vi "TCP-IP Q_Bridge.Core.vi"(4 "Notification":bool, 6 "Auto Exit":bool, 7 "StatusCtrlRef":refnum<vi>, 8 "Config":T1={"IP"="127.0.0.1", "Port"=8500, "Listener"=FALSE, "Enable"=FALSE}, 9 "Q_DataOut":refnum<queue> caption="Q_DataOut(To TCP-IP)", 10 "Q_DataIn":refnum<queue> caption="Q_DataIn(From TCP-IP)", 11 "Control Q":string="TCP-IP_Bridge") -> ()   [LabVIEW 2024, in "EQMF.lvlib" / "TCP-IP.lvlib"]
uses:
  TCP-IP.lvlib
  Queues/Q.Element.ctl
  Mgr/TCP-IP Mgr.Config.ctl
  Queues/Queue Utils.lvlib
panel:
  out "Close":bool
  out "connection ID":refnum<k5>
  out "listener ID":refnum<k5>
  out "Exit":bool
  out "Connected":bool
  out "error out":errorcluster
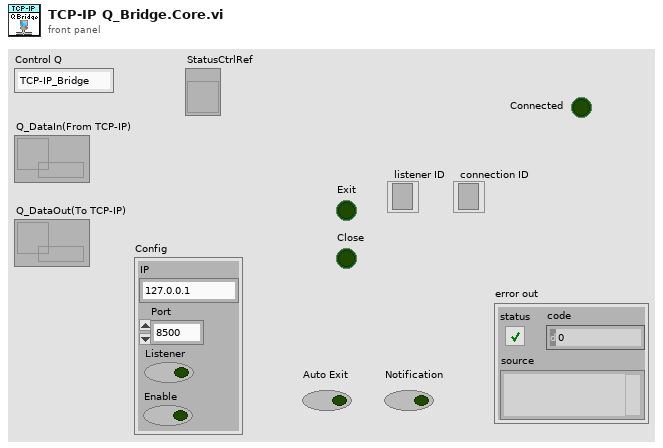
[diagram p1: front panel]
types:
  T1 = typedef "EQMF.lvlib/TCP-IP.lvlib/TCP-IP Mgr.Config.ctl" = cluster{"IP":string, "Port":u16, "Listener":bool, "Enable":bool}
  T2 = typedef "EQMF.lvlib/Queue Utils.lvlib/Q.Element.ctl" = cluster{"Cmd":string, "Sub":string, "Data1":variant, "Data2":variant}
  T3 = cluster{"Config":T1, "ConnectionID":refnum<k5>, "listenerID":refnum<k5>, "Connected":bool, "StatusCtrlRef":refnum<vi>, "CtrlRefEn":bool}
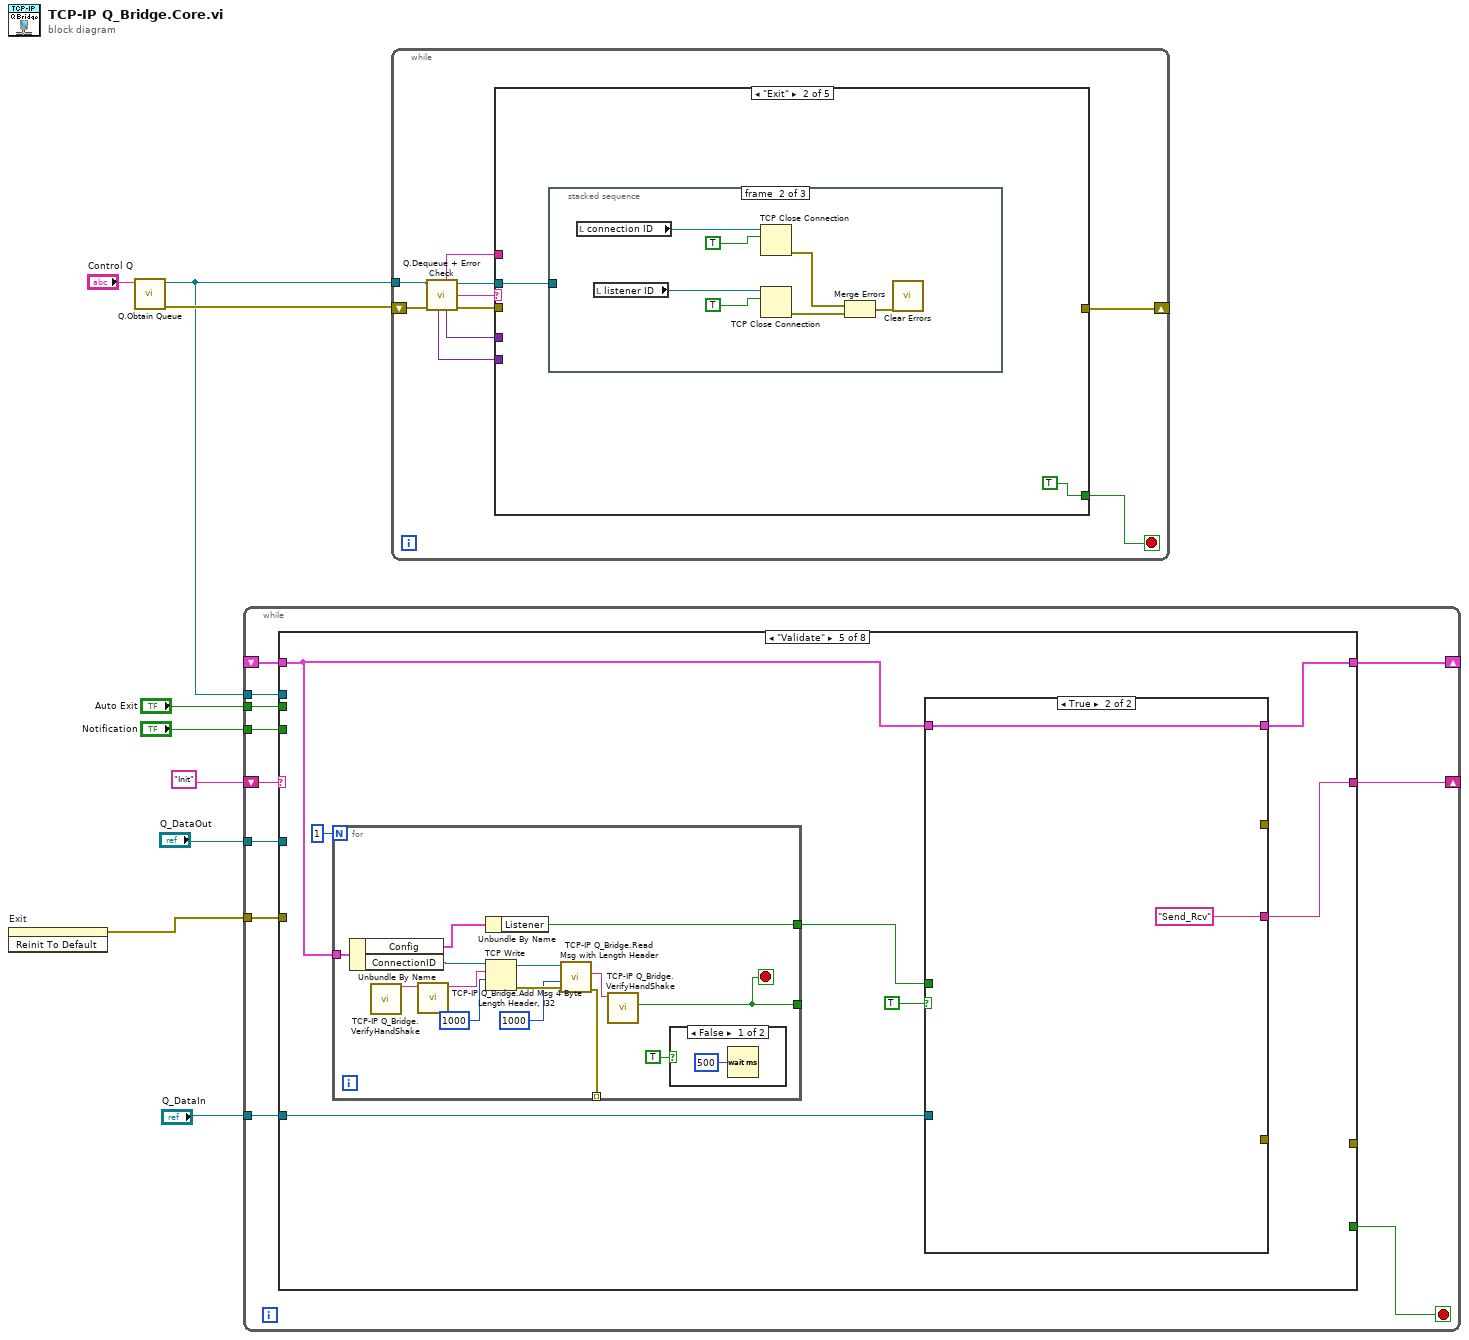
[diagram p0: block diagram]
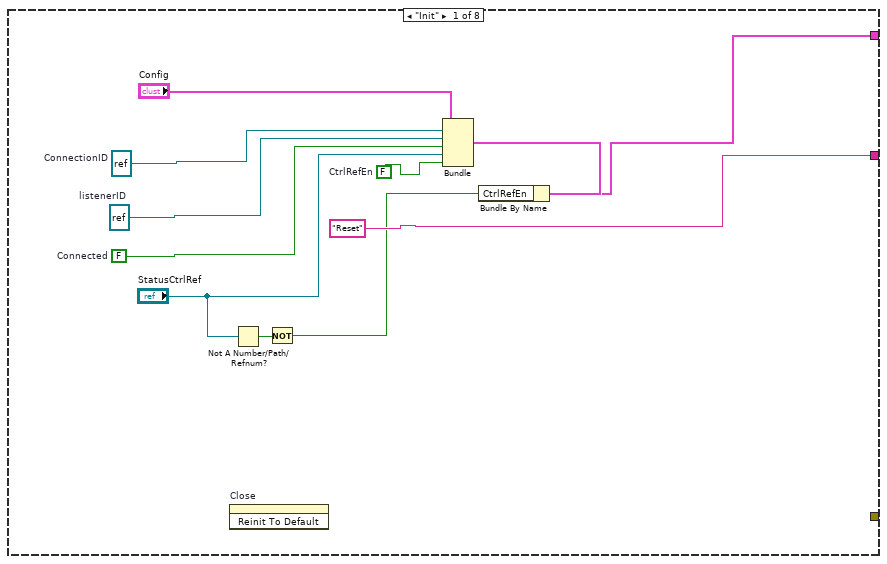
[diagram p2: hidden frame]
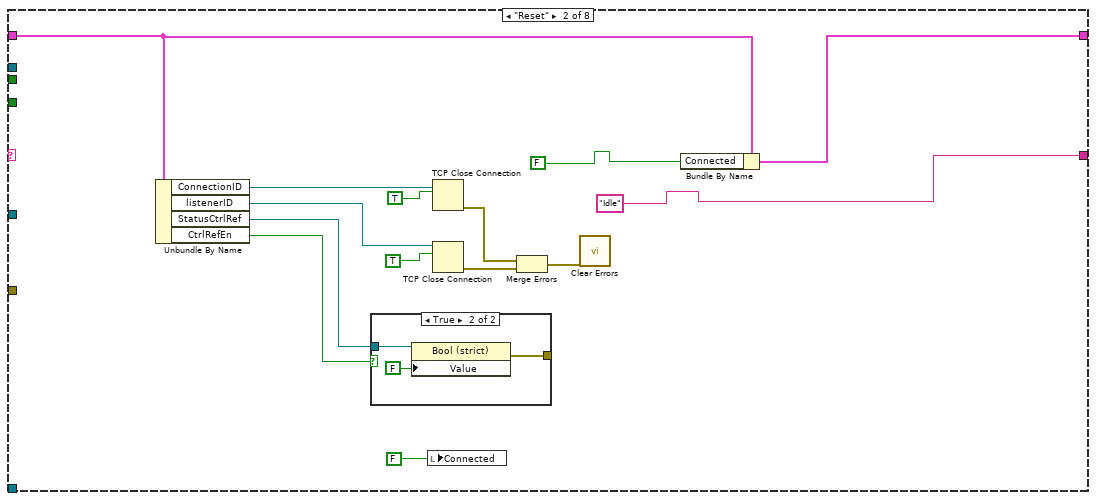
[diagram p3: hidden frame]
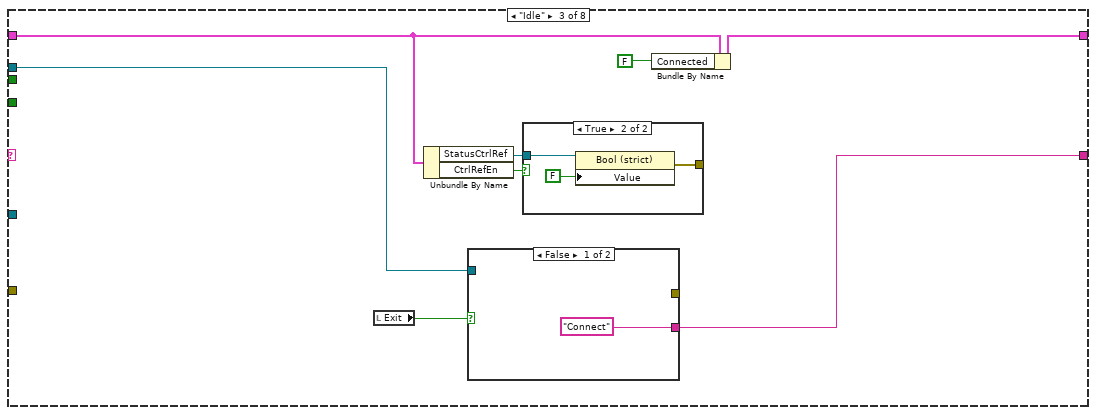
[diagram p5: hidden frame]
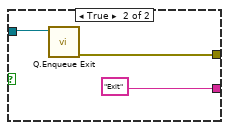
[diagram p7: hidden frame]
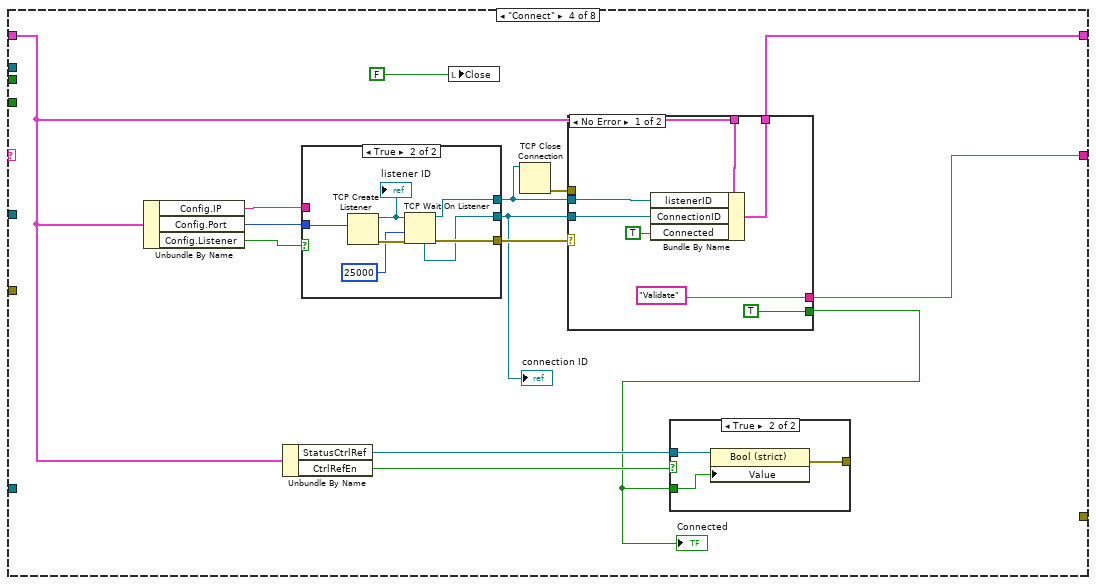
[diagram p8: hidden frame]
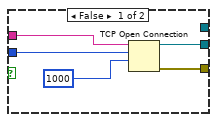
[diagram p10: hidden frame]
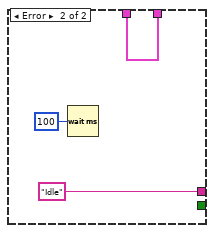
[diagram p11: hidden frame]
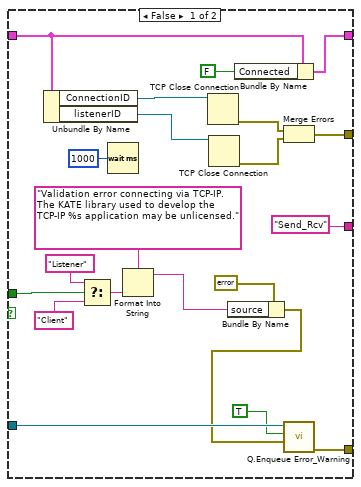
[diagram p13: hidden frame]
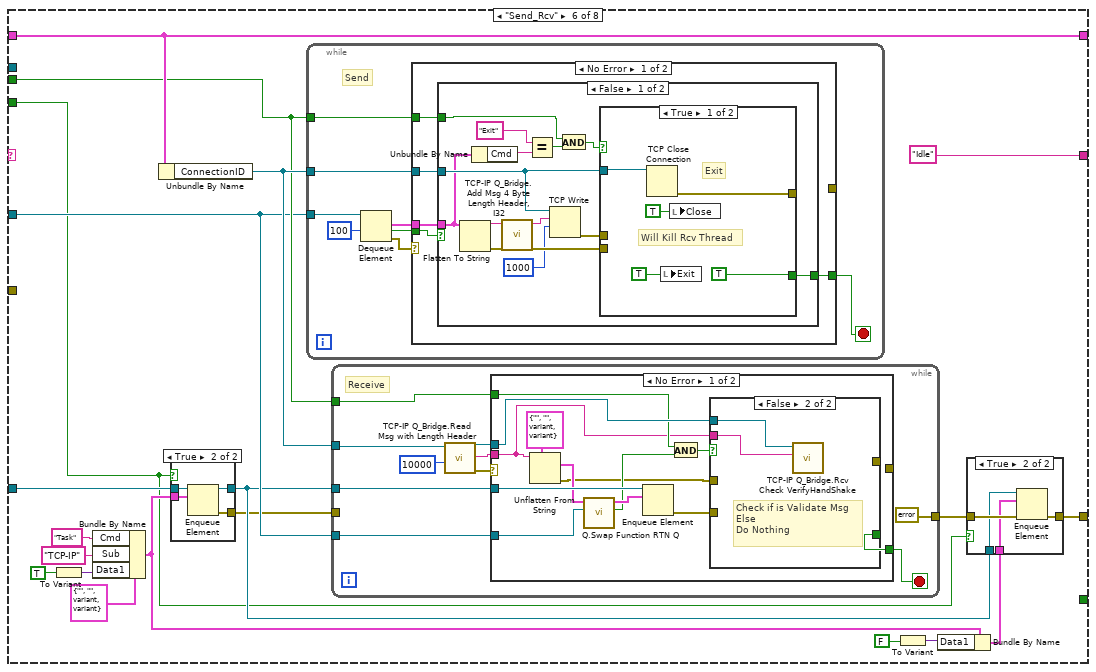
[diagram p14: hidden frame]
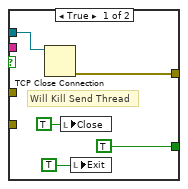
[diagram p17: hidden frame]
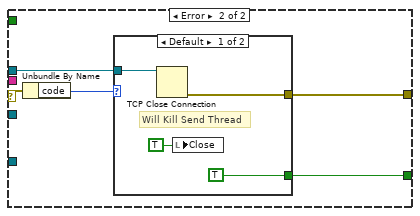
[diagram p18: hidden frame]
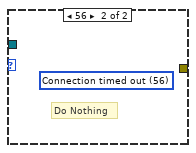
[diagram p19: hidden frame]
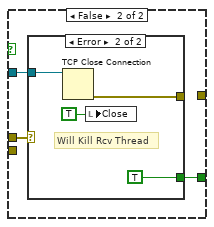
[diagram p20: hidden frame]
diagram:
  n1 = invoke on="Exit" class="Bool (strict)" method="Reinit To Default"() -> (error out=w4:errorcluster)  [unwired: 3 in, 2 out]
  n2 = call "Q.Obtain Queue.vi"("Q Name"="Control Q") -> ("error out"=w8:errorcluster, "Q Out"=w3:refnum<queue>)  [unwired: 8 in, 1 out]
  n3 = while {
    shift-right: [w18] -> _
    shift-left: _ -> [w19]
    shift-right: [w13] -> _
    shift-left: "Init" -> [w20]
    tunnel: "Q_DataOut" -> [w16]
    tunnel: "Q_DataIn" -> [w15]
    tunnel: w4 -> [w14]
    tunnel: w3 -> [w12]
    tunnel: "Auto Exit" -> [w11]
    tunnel: "Notification" -> [w10]
    stop <- w17 stop-if-true
    n4 = case shown="\"Validate\"" w20 {
      tunnel: w19 -> [_ w38 w51 w70 w107 w167 w262 w270]
      tunnel: [w22 w37 w56 w75 w106 w167 w262 w270] -> w18
      tunnel: ["Reset" "Idle" w54 w74 w109 "Idle" "Reset" "Exit"] -> w13
      tunnel: [_ _ _ _ _ _ _ TRUE] -> w17
      tunnel: w16 -> [_ _ _ _ _ w163 _ _]
      tunnel: w15 -> [_ _ _ _ w105 w157 _ _]
      tunnel: w14 -> [_ _ _ _ _ _ _ _]
      tunnel: w12 -> [_ _ w52 _ _ _ _ w265]
      tunnel: w11 -> [_ _ _ _ _ w164 _ _]
      tunnel: w10 -> [_ _ _ _ _ w148 _ _]
      tunnel: [_ _ _ _ _ w155 _ _] -> _
      frame "Init" {
        w24 = FALSE  # CtrlRefEn
        w27 = FALSE  # Connected
        w28 = refnum<k5> refnum  # listenerID
        w29 = refnum<k5> refnum  # ConnectionID
        n5 = invoke on="Close" class="Bool (strict)" method="Reinit To Default"() -> ()  [unwired: 3 in, 3 out]
        n6 = Not A Number/Path/Refnum?(number/path/refnum="StatusCtrlRef") -> (NaN/Path/Refnum?=w25:bool)
        n7 = Not(x=w25) -> (.not. x?=w21:bool)
        n8 = Bundle("Config"="Config", "ConnectionID"=w29, "listenerID"=w28, "Connected"=w27, "StatusCtrlRef"="StatusCtrlRef", "CtrlRefEn"=w24) -> (w23:T3)  [unwired: 1 in]
        n9 = Bundle By Name(cluster=w23, "CtrlRefEn"=w21) -> (w22:T3)
      }
      frame "Reset" {
        n10 = Unbundle By Name(w38) -> ("ConnectionID"=w45:refnum<k5>, "listenerID"=w42:refnum<k5>, "StatusCtrlRef"=w34:refnum<vi>, "CtrlRefEn"=w33:bool)
        n11 = case shown="True" w33 {
          tunnel: w34 -> [_ w48]
          tunnel: [_ w46] -> _
          frame False {
          }
          frame True {
            n12 = property class="Bool (strict)"(reference=w48, "Value"=FALSE) -> (error out=w46:errorcluster)  [unwired: 1 in, 1 out]
          }
        }
        n13 = local write "Connected"(FALSE ("Value")) -> ()
        n14 = TCP Close Connection(connection ID=w45, abort (F)=TRUE) -> (error out=w40:errorcluster)  [unwired: 1 in, 1 out]
        n15 = TCP Close Connection(connection ID=w42, abort (F)=TRUE) -> (error out=w41:errorcluster)  [unwired: 1 in, 1 out]
        n16 = Merge Errors(w40, w41) -> (w39:errorcluster)
        n17 = call <vilib>:"Clear Errors.vi"("error in (no error)"=w39) -> ()  [unwired: 5 in, 2 out]
        n18 = Bundle By Name(cluster=w38, "Connected"=FALSE) -> (w37:T3)
      }
      frame "Idle" {
        n19 = local read "Exit"() -> (w53:bool)
        n20 = Unbundle By Name(w51) -> ("StatusCtrlRef"=w50:refnum<vi>, "CtrlRefEn"=w49:bool)
        n21 = case shown="False" w53 {
          tunnel: ["Connect" "Exit"] -> w54
          tunnel: w52 -> [_ w62]
          tunnel: [_ w61] -> _
          frame False {
          }
          frame True {
            n22 = call "Q.Enqueue Exit.vi"("Q In"=w62) -> ("error out"=w61:errorcluster)  [unwired: 9 in, 1 out]
          }
        }
        n23 = case shown="True" w49 {
          tunnel: w50 -> [_ w59]
          tunnel: [_ w58] -> _
          frame False {
          }
          frame True {
            n24 = property class="Bool (strict)"(reference=w59, "Value"=FALSE ("Connected")) -> (error out=w58:errorcluster)  [unwired: 1 in, 1 out]
          }
        }
        n25 = Bundle By Name(cluster=w51, "Connected"=FALSE) -> (w56:T3)
      }
      frame "Connect" {
        n26 = Unbundle By Name(w70) -> ("Config.IP"=w77:string, "Config.Port"=w76:u16, "Config.Listener"=w72:bool)
        n27 = Unbundle By Name(w70) -> ("StatusCtrlRef"=w69:refnum<vi>, "CtrlRefEn"=w68:bool)
        n28 = case shown="True" w72 {
          tunnel: w77 -> [w85 _]
          tunnel: w76 -> [w84 w92]
          tunnel: [w82 w87] -> w71
          tunnel: [w81 w89] -> w73
          tunnel: [_ w88] -> w65
          frame False {
            n29 = TCP Open Connection(address=w85, remote port or service name=w84, timeout ms (60000)=1000) -> (connection ID=w82:refnum<k5>, error out=w81:errorcluster)  [unwired: 2 in]
          }
          frame True {
            n30 = TCP Create Listener(10:w92) -> (0:w91:errorcluster, 3:w90:refnum<k5>)  [unwired: 4 in, 1 out]
            "listener ID" <- w90
            n31 = TCP Wait On Listener(8:w91, 9:25000 ("timeout ms (wait forever: -1)"), 11:w90) -> (0:w89:errorcluster, 3:w88:refnum<k5>, 4:w87:refnum<k5>)  [unwired: 1 in, 2 out]
          }
        }
        "connection ID" <- w71
        n32 = local write "Close"(FALSE ("Reset")) -> ()
        n33 = TCP Close Connection(connection ID=w65) -> (error out=w64:errorcluster)  [unwired: 2 in, 1 out]
        n34 = case shown="No Error" w73 {
          tunnel: w70 -> [w99 w100]
          tunnel: w71 -> [w97 _]
          tunnel: [w96 w100] -> w75
          tunnel: ["Validate" "Idle"] -> w74
          tunnel: w65 -> [w93 _]
          tunnel: [TRUE _] -> w67
          tunnel: w64 -> [_ _]
          frame No Error {
            n35 = Bundle By Name(cluster=w99, "listenerID"=w93, "ConnectionID"=w97, "Connected"=TRUE) -> (w96:T3)
          }
          frame Error {
            n36 = Wait (ms)(milliseconds to wait=u32 100) -> ()  [unwired: 1 out]
          }
        }
        "Connected" <- w67
        n37 = case shown="True" w68 {
          tunnel: w69 -> [_ w80]
          tunnel: [_ w79] -> _
          tunnel: w67 -> [_ w78]
          frame False {
          }
          frame True {
            n38 = property class="Bool (strict)"(reference=w80, "Value"=w78) -> (error out=w79:errorcluster)  [unwired: 1 in, 1 out]
          }
        }
      }
      frame "Validate" {
        n39 = for {
          N: 1 -> [_]
          tunnel: [w112] -> _
          tunnel: [w114] -> w108
          tunnel: w107 -> [w113]
          tunnel: [w111] -> _ mode=indexing
          stop <- w112 stop-if-true
          n40 = Unbundle By Name(w113) -> ("Config"=w115:T1, "ConnectionID"=w122:refnum<k5>)
          n41 = call "TCP-IP Q_Bridge.VerifyHandShake.vi"() -> ("Msg Out"=w117:string)  [unwired: 10 in, 1 out]
          n42 = call "TCP-IP Q_Bridge.Add Msg 4 Byte Length Header, I32.vi"("Message"=w117) -> ("Message + Header"=w123:string)  [unwired: 10 in]
          n43 = Unbundle By Name(w115) -> ("Listener"=w114:bool)
          n44 = TCP Write(connection ID=w122, data in=w123, 9:1000 ("timeout ms (25000)")) -> (connection ID out=w121:refnum<k5>, error out=w120:errorcluster)  [unwired: 1 in, 1 out]
          n45 = call "TCP-IP Q_Bridge.Read Msg with Length Header.vi"("error in (no error)"=w120, "Timeoutms"=1000 ("timeout ms (25000)"), "ConID"=w121) -> ("Error Out"=w111:errorcluster, "data out"=w116:string)  [unwired: 5 in, 2 out]
          n46 = call "TCP-IP Q_Bridge.VerifyHandShake.vi"("Msg In"=w116) -> ("OK"=w112:bool)  [unwired: 9 in, 1 out]
          n47 = case shown="False" TRUE {
            frame False {
              n48 = Wait (ms)(milliseconds to wait=u32 500) -> ()  [unwired: 1 out]
            }
            frame True {
            }
          }
        }
        n49 = case shown="True" TRUE {
          tunnel: ["Send_Rcv" "Send_Rcv"] -> w109
          tunnel: w108 -> [w142 _]
          tunnel: w107 -> [w136 w146]
          tunnel: [w137 w146] -> w106
          tunnel: [w131 _] -> _
          tunnel: w105 -> [w130 _]
          tunnel: [w125 _] -> _
          frame False {
            n50 = Unbundle By Name(w136) -> ("ConnectionID"=w135:refnum<k5>, "listenerID"=w134:refnum<k5>)
            n51 = Select(t="Listener", s=w142, f="Client") -> (s? t:f=w143:string)
            n52 = Wait (ms)(milliseconds to wait=u32 1000) -> ()  [unwired: 1 out]
            n53 = Format Into String(format string="Validation error connecting via TCP-IP.  The KATE library used to develop the TCP-IP %s application may be unlicensed." ("message"), w143) -> (resulting string=w128:string)  [unwired: 2 in, 1 out]
            n54 = TCP Close Connection(connection ID=w135) -> (error out=w133:errorcluster)  [unwired: 2 in, 1 out]
            n55 = TCP Close Connection(connection ID=w134) -> (error out=w132:errorcluster)  [unwired: 2 in, 1 out]
            n56 = Bundle By Name(cluster=errorcluster {"status"=TRUE, "code"=-8000, "source"=""} ("error constant"), "source"=w128) -> (w127:errorcluster)
            n57 = Bundle By Name(cluster=w136, "Connected"=FALSE) -> (w137:T3)
            n58 = Merge Errors(w133, w132) -> (w131:errorcluster)
            n59 = call "Q.Enqueue Error_Warning.vi"("Error/Warning"=w127, "Warning(F)/Error(T)"=TRUE, "Q In"=w130) -> ("error out"=w125:errorcluster)  [unwired: 7 in, 1 out]
          }
          frame True {
          }
        }
      }
      frame "Send_Rcv" {
        n60 = To Variant(anything=TRUE) -> (Variant=w161:variant)
        n61 = Bundle By Name(cluster=T2 {"Cmd"="", "Sub"="", "Data1"=variant, "Data2"=variant} ("Q.Element"), "Cmd"="Task", "Sub"="TCP-IP", "Data1"=w161) -> (w151:T2)
        n62 = Unbundle By Name(w167) -> ("ConnectionID"=w166:refnum<k5>)
        n63 = case shown="True" w148 {
          tunnel: w157 -> [w172 w176]
          tunnel: [w172 w175] -> w154
          tunnel: w151 -> [_ w174]
          tunnel: [_ w173] -> w149
          frame False {
          }
          frame True {
            n64 = Enqueue Element(queue=w176, element=w174) -> (queue out=w175:refnum<queue>, error out=w173:errorcluster)  [unwired: 2 in, 1 out]
          }
        }
        n65 = while {
          tunnel: w163 -> [w222]
          tunnel: w166 -> [w220]
          tunnel: w164 -> [w217]
          stop <- w223 stop-if-true
          # "Send"
          n66 = Dequeue Element(queue=w222, timeout in ms (-1)=100) -> (element=w218:T2, timed out?=w219:bool, error out=w216:errorcluster)  [unwired: 1 in, 1 out]
          n67 = case shown="No Error" w216 {
            tunnel: [w228 TRUE] -> w223
            tunnel: w220 -> [w227 w257]
            tunnel: w219 -> [w226 _]
            tunnel: w218 -> [w225 _]
            tunnel: w217 -> [w224 _]
            tunnel: [_ w256] -> _
            frame No Error {
              n68 = case shown="False" w226 {
                tunnel: [w241 w254] -> w228
                tunnel: w225 -> [w238 _]
                tunnel: w227 -> [w240 _]
                tunnel: w224 -> [w233 _]
                frame False {
                  n69 = Flatten To String(anything=w238) -> (data string=w232:string, error out=w230:errorcluster)  [unwired: 3 in, 1 out]
                  n70 = Unbundle By Name(w238) -> ("Cmd"=w237:string)
                  n71 = call "TCP-IP Q_Bridge.Add Msg 4 Byte Length Header, I32.vi"("Message"=w232) -> ("Message + Header"=w231:string)  [unwired: 10 in]
                  n72 = Equal?(x="Exit", y=w237) -> (x = y?=w235:bool)
                  n73 = TCP Write(connection ID=w240, data in=w231, 9:1000 ("timeout ms (25000)")) -> (error out=w239:errorcluster)  [unwired: 1 in, 2 out]
                  n74 = And(x=w233, y=w235) -> (x .and. y?=w234:bool)
                  n75 = case shown="True" w234 {
                    tunnel: [TRUE w249] -> w241
                    tunnel: w240 -> [w245 w248]
                    tunnel: w239 -> [_ w247]
                    tunnel: [w244 _] -> _
                    tunnel: w230 -> [_ _]
                    frame True {
                      # "Exit"
                      # "Will Kill Rcv Thread"
                      n76 = TCP Close Connection(connection ID=w245) -> (error out=w244:errorcluster)  [unwired: 2 in, 1 out]
                      n77 = local write "Exit"(TRUE ("Close")) -> ()
                      n78 = local write "Close"(TRUE ("Close")) -> ()
                    }
                    frame False {
                      n79 = case shown="Error" w247 {
                        tunnel: w248 -> [_ w252]
                        tunnel: [_ TRUE] -> w249
                        tunnel: [_ w251] -> _
                        frame No Error {
                        }
                        frame Error {
                          # "Will Kill Rcv Thread"
                          n80 = TCP Close Connection(connection ID=w252) -> (error out=w251:errorcluster)  [unwired: 2 in, 1 out]
                          n81 = local write "Close"(TRUE ("Close")) -> ()
                        }
                      }
                    }
                  }
                }
                frame True {
                  # "This time out allows ability to stop/exit"
                  # "Do nothing\nTimed Out"
                  n82 = local read "Close"() -> (w254:bool)
                }
              }
            }
            frame Error {
              # "Exit"
              # "Will Kill Rcv Thread"
              n83 = TCP Close Connection(connection ID=w257) -> (error out=w256:errorcluster)  [unwired: 2 in, 1 out]
              n84 = local write "Exit"(TRUE ("Close")) -> ()
              n85 = local write "Close"(TRUE ("Close")) -> ()
            }
          }
        }
        n86 = while {
          tunnel: w154 -> [w186]
          tunnel: w166 -> [w181]
          tunnel: w164 -> [w184]
          tunnel: w163 -> [w183]
          tunnel: [errorcluster {"status"=FALSE, "code"=0, "source"=""} ("error constant")] -> w156
          tunnel: w149 -> [_]
          stop <- w185 stop-if-true
          # "Receive"
          n87 = call "TCP-IP Q_Bridge.Read Msg with Length Header.vi"("Timeoutms"=10000 ("timeout ms (25000)"), "ConID"=w181) -> ("Error Out"=w178:errorcluster, "data out"=w179:string, "ConID Out"=w182:refnum<k5>)  [unwired: 6 in, 1 out]
          n88 = case shown="No Error" w178 {
            selector: w178 -> [_ w208]
            tunnel: w186 -> [w198 _]
            tunnel: w182 -> [w197 w210]
            tunnel: [w196 w211] -> w185
            tunnel: [_ w209] -> _
            tunnel: w184 -> [w194 _]
            tunnel: w183 -> [w190 _]
            tunnel: w179 -> [w187 _]
            frame No Error {
              n89 = Unflatten From String(type=T2 {"Cmd"="", "Sub"="", "Data1"=variant, "Data2"=variant} ("Q.Element"), binary string=w187) -> (value=w193:T2, error out=w189:errorcluster)  [unwired: 3 in, 1 out]
              n90 = call "Q.Swap Function RTN Q.vi"("RtnQ In"=w190, "Q.Element"=w193) -> ("Exit"=w191:bool, "Q.Element Out"=w192:T2)  [unwired: 8 in]
              n91 = Enqueue Element(queue=w198, element=w192) -> (error out=w188:errorcluster)  [unwired: 2 in, 2 out]
              n92 = And(x=w194, y=w191) -> (x .and. y?=w195:bool)
              n93 = case shown="False" w195 {
                tunnel: [TRUE _] -> w196
                tunnel: w197 -> [w203 w206]
                tunnel: [w202 _] -> _
                tunnel: w189 -> [_ _]
                tunnel: w188 -> [_ _]
                tunnel: w187 -> [_ w205]
                frame True {
                  # "Will Kill Send Thread"
                  n94 = TCP Close Connection(connection ID=w203) -> (error out=w202:errorcluster)  [unwired: 2 in, 1 out]
                  n95 = local write "Close"(TRUE ("Close")) -> ()
                  n96 = local write "Exit"(TRUE ("Close")) -> ()
                }
                frame False {
                  # "Check if is Validate Msg\nElse\nDo Nothing"
                  n97 = call "TCP-IP Q_Bridge.Rcv Check VerifyHandShake.vi"("Msg In"=w205, "ConID"=w206) -> ()  [unwired: 7 in, 3 out]
                }
              }
            }
            frame Error {
              n98 = Unbundle By Name(w208) -> ("code"=w207:i32)
              n99 = case shown="Default" w207 {
                tunnel: [TRUE _] -> w211
                tunnel: w210 -> [w214 _]
                tunnel: [w213 _] -> w209
                frame Default {
                  # "Will Kill Send Thread"
                  n100 = TCP Close Connection(connection ID=w214) -> (error out=w213:errorcluster)  [unwired: 2 in, 1 out]
                  n101 = local write "Close"(TRUE ("Close")) -> ()
                }
                frame 56 {
                  (unwired) 56 items=["No Error", "Argument Error", "Memory Full", "Out of Zone", "End of File", "File Already Open", "Generic File IO Error", "File Not Found", "File Permission Error", "Disk Full", "Duplicate Path", "Too Many Files Open", "Not Enabled", "Resource File Not Found", "Cannot Add Resource", "Resource Not Found", "Image Not Found", "Image Memory Error", "Pen Does Not Exist", "Config Bad Type", "Config Token Not Found", "Config Parse Error", "Config Memory Error", "Bad External Code Format", "Bad External Code Offset", "External Code Not Present", "Null Window", "Destroy Window Mixup", "Null Menu", "Print Aborted", "Bad Print Record", "Print Driver Error", "Windows Error During Print", "Memory Error During Print", "Print Dialog Error", "Generic Print Error", "Invalid Device Refnum", "Device Not Found", "Device Parameter Error", "Device Unit Error", "Can't Open Device", "Device Call Aborted", "Generic Error", "Cancelled By User", "Object ID Too Low", "Object ID Too High", "Object Not In Heap", "Unknown Heap", "Bad DefProc ID", "DefProc Not In Table", "Message Out Of Range", "Null Method", "Unknown Message", "Manager Call Not Supported", "Bad address", "Connection In progress", "Connection timed out", "Connection is already in progress", "Network attribute not supported", "Network error", "Address in use", "System out of memory", "Connection aborted", "Connection refused", "Connection is not connected", "Connection is already connected", "Connection closed", "Initialize error (interapplication manager)", "Bad occurrence", "Wait on unbound occurrence handler", "Occurrence queue overflow", "Bad path", "Semaphore not signaled", "Unrecognized type (interapplication manager)"] ("2nd Error to Convert")
                  # "Do Nothing"
                }
              }
            }
          }
        }
        n102 = To Variant(anything=FALSE) -> (Variant=w153:variant)
        n103 = Bundle By Name(cluster=w151, "Data1"=w153) -> (w150:T2)
        n104 = case shown="True" w148 {
          tunnel: w156 -> [_ w171]
          tunnel: [_ w170] -> w155
          tunnel: w154 -> [_ w169]
          tunnel: w150 -> [_ w168]
          frame False {
          }
          frame True {
            n105 = Enqueue Element(queue=w169, element=w168, error in (no error)=w171) -> (error out=w170:errorcluster)  [unwired: 1 in, 2 out]
          }
        }
      }
      frame "Error", Default {
        n106 = Wait (ms)(milliseconds to wait=u32 100) -> ()  [unwired: 1 out]
      }
      frame "Exit" {
        n107 = Unbundle By Name(w270) -> ("ConnectionID"=w272:refnum<k5>, "listenerID"=w271:refnum<k5>, "StatusCtrlRef"=w268:refnum<vi>, "CtrlRefEn"=w267:bool)
        n108 = Not A Number/Path/Refnum?(number/path/refnum=w265) -> (NaN/Path/Refnum?=w264:bool)
        n109 = case shown="True" w267 {
          tunnel: w268 -> [_ w285]
          tunnel: [_ w283] -> _
          frame False {
          }
          frame True {
            n110 = property class="Bool (strict)"(reference=w285, "Value"=FALSE) -> (error out=w283:errorcluster)  [unwired: 1 in, 1 out]
          }
        }
        n111 = case shown="True" TRUE {
          tunnel: w272 -> [_ w280]
          tunnel: w271 -> [_ w277]
          frame False {
          }
          frame True {
            n112 = TCP Close Connection(connection ID=w280, abort (F)=TRUE) -> (error out=w275:errorcluster)  [unwired: 1 in, 1 out]
            n113 = TCP Close Connection(connection ID=w277, abort (F)=TRUE) -> (error out=w276:errorcluster)  [unwired: 1 in, 1 out]
            n114 = Merge Errors(w275, w276) -> (w274:errorcluster)
            n115 = call <vilib>:"Clear Errors.vi"("error in (no error)"=w274) -> ()  [unwired: 5 in, 2 out]
          }
        }
        n116 = local write "Connected"(FALSE ("Value")) -> ()
        n117 = case shown="False" w264 {
          tunnel: w265 -> [w281 _]
          frame False {
            n118 = call "Q.Enqueue Exit.vi"("Q In"=w281) -> ("error out"=w282:errorcluster)  [unwired: 9 in, 1 out]
            n119 = call <vilib>:"Clear Errors.vi"("error in (no error)"=w282) -> ()  [unwired: 5 in, 2 out]
          }
          frame True {
          }
        }
      }
    }
  }
  n120 = while {
    tunnel: w3 -> [w295]
    shift-right: [w287] -> _
    shift-left: w8 -> [w294]
    stop <- w286 stop-if-true
    n121 = call "Q.Dequeue + Error Check.vi"("Error In"=w294, "Q In"=w295) -> ("error out"=w291:errorcluster, "Cmd"=w293:string, "Q Out"=w292:refnum<queue>, "Data1"=w290:variant, "Sub"=w288:string, "Data2"=w289:variant)  [unwired: 4 in]
    n122 = case shown="\"Exit\"" w293 {
      tunnel: w292 -> [_ w305 _ _ w325]
      tunnel: w291 -> [w299 _ _ _ w326]
      tunnel: w290 -> [w297 _ _ _ w327]
      tunnel: w289 -> [_ _ _ _ _]
      tunnel: w288 -> [w300 _ _ _ w328]
      tunnel: [errorcluster {"status"=FALSE, "code"=0, "source"=""} ("error constant") _ _ _ _] -> w287
      tunnel: [_ TRUE _ _ _] -> w286
      frame "Error", Default {
        n123 = case shown="\"Clear\", Default" w300 {
          tunnel: w299 -> [_ w304]
          tunnel: [w302 w304] -> w298
          tunnel: w297 -> [w301 _]
          frame "Error" {
            n124 = Variant To Data(type=errorcluster {"status"=FALSE, "code"=0, "source"=""} ("error constant"), Variant=w301) -> (data=w302:errorcluster)  [unwired: 1 in, 1 out]
          }
          frame "Clear", Default {
          }
        }
        "error out" <- w298
      }
      frame "Exit" {
        n125 = stacked-sequence {
          tunnel: w305 -> [_ _ w316]
          frame #0 {
            n126 = local write "Close"(TRUE ("Reset")) -> ()
            "Exit" <- TRUE ("Exit")
          }
          frame #1 {
            n127 = local read "connection ID"() -> (w310:refnum<k5>)
            n128 = local read "listener ID"() -> (w309:refnum<k5>)
            n129 = TCP Close Connection(connection ID=w310, abort (F)=TRUE) -> (error out=w314:errorcluster)  [unwired: 1 in, 1 out]
            n130 = TCP Close Connection(connection ID=w309, abort (F)=TRUE) -> (error out=w313:errorcluster)  [unwired: 1 in, 1 out]
            n131 = Merge Errors(w314, w313) -> (w315:errorcluster)
            n132 = call <vilib>:"Clear Errors.vi"("error in (no error)"=w315) -> ()  [unwired: 5 in, 2 out]
          }
          frame #2 {
            n133 = Release Queue(queue=w316) -> ()  [unwired: 2 in, 3 out]
          }
        }
      }
      frame "Init" {
      }
      frame "Reset" {
        n134 = local read "connection ID"() -> (w320:refnum<k5>)
        n135 = local read "listener ID"() -> (w319:refnum<k5>)
        n136 = TCP Close Connection(connection ID=w320, abort (F)=TRUE) -> (error out=w322:errorcluster)  [unwired: 1 in, 1 out]
        n137 = TCP Close Connection(connection ID=w319, abort (F)=TRUE) -> (error out=w321:errorcluster)  [unwired: 1 in, 1 out]
        n138 = Merge Errors(w322, w321) -> (w323:errorcluster)
        n139 = call <vilib>:"Clear Errors.vi"("error in (no error)"=w323) -> ()  [unwired: 5 in, 2 out]
        "Close" <- TRUE ("Reset")
      }
      frame "Task" {
        n140 = case shown="\"True\"" w328 {
          tunnel: w327 -> [_ _]
          tunnel: w326 -> [_ _]
          tunnel: w325 -> [_ _]
          frame Default {
          }
          frame "True" {
          }
        }
      }
    }
  }
